vi "BRig_dataExp_T_Selection.vi"() -> (2 "output_T_Selection":i32)   [LabVIEW 2014]
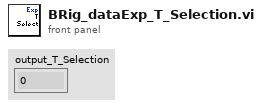
[diagram p1: front panel]
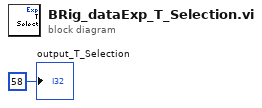
[diagram p0: block diagram]
diagram:
  "output_T_Selection" <- 58 ("output_iBlock")
